vi "Write.vi"(8 "error in (no error)":errorcluster, 11 "VeriStand DSF in":refnum<class "VeriStand DSF.lvclass">=refnum) -> (0 "error out":errorcluster, 3 "VeriStand DSF out":refnum<class "VeriStand DSF.lvclass">)   [LabVIEW 2019, in "DSF Engine.lvlib" / "VeriStand DSF.lvclass"]
uses:
  VeriStand DSF.lvclass
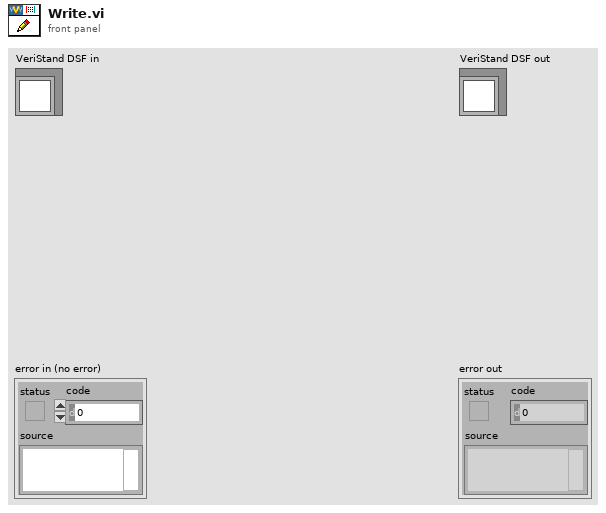
[diagram p1: front panel]
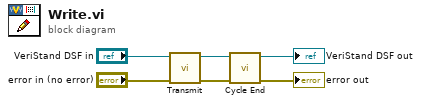
[diagram p0: block diagram]
diagram:
  n1 = call "Transmit.vi"("error in"="error in (no error)", "framework in"="VeriStand DSF in") -> ("error out"=w5:errorcluster, "framework out"=w6:refnum<class "VeriStand DSF.lvclass">)  [unwired: 8 in]
  n2 = call "Cycle End.vi"("error in (no error)"=w5, "Framework in"=w6) -> ("error out"=→"error out":errorcluster, "Framework out"=→"VeriStand DSF out":refnum<class "VeriStand DSF.lvclass">)  [unwired: 8 in]
